vi "HFRR ADV v09 new software.vi"() -> ()   [LabVIEW 2025] (continued)
            n3576 = local read "SEN.RUN HRS"() -> (w4464:dbl)
            n3577 = Divide(x=w4468, y=w4476) -> (x/y=w4475:dbl)
            n3578 = Increment(x=w4475) -> (x+1=w4471:dbl)
            n3579 = Number To Decimal String(number=w4471) -> (decimal integer string=→"run hrs":string)  [unwired: 1 in]
            n3580 = Divide(x=w4464, y=3600.0 ("f")) -> (x/y=w4459:dbl)
            n3581 = Round To Nearest(number=w4459) -> (nearest integer value=w4457:dbl)
            n3582 = Number To Decimal String(number=w4457) -> (decimal integer string=w4458:string)  [unwired: 1 in]
            n3583 = Number To Decimal String(number=w4466) -> (decimal integer string=w4467:string)  [unwired: 1 in]
            n3584 = local read "Model No"() -> (w4472:string)
            n3585 = local read "UUID"() -> (w4567:string)
            n3586 = local read "Serial No"() -> (w4571:string)
            n3587 = local read "Secret Key"() -> (w4572:string)
            n3588 = Concatenate Strings("\",\"MachineSerialNumber\":\"" ("string"), w4571) -> (w4575:string)
            n3589 = Concatenate Strings("\",\"ModelNumber\":\"" ("string"), w4472) -> (w4473:string)
            n3590 = Concatenate Strings("\",\"MachineRuntimeHours\":\"" ("string"), w4458) -> (w4576:string)
            n3591 = Concatenate Strings("\",\"MachineRuntimeCycles\":\"", w4467) -> (w4569:string)
            n3592 = Concatenate Strings(w4525, w4521) -> (w4555:string)
            n3593 = Concatenate Strings(w4524, w4511) -> (w4556:string)
            n3594 = Concatenate Strings(w4523, w4493) -> (w4554:string)
            n3595 = Concatenate Strings(w4575, w4473, w4576, w4569) -> (w4578:string)
            n3596 = Concatenate Strings(w4525, w4520) -> (w4552:string)
            n3597 = Concatenate Strings(w4524, w4510) -> (w4551:string)
            n3598 = Concatenate Strings(w4523, w4492) -> (w4553:string)
            n3599 = Concatenate Strings(w4525, w4519) -> (w4547:string)
            n3600 = Concatenate Strings(w4524, w4509) -> (w4548:string)
            n3601 = Concatenate Strings(w4523, w4491) -> (w4546:string)
            n3602 = Concatenate Strings(w4525, w4518) -> (w4544:string)
            n3603 = Concatenate Strings(w4524, w4508) -> (w4543:string)
            n3604 = Concatenate Strings(w4523, w4490) -> (w4545:string)
            n3605 = Concatenate Strings(w4555, w4556, w4554) -> (w4557:string)
            n3606 = Concatenate Strings(w4525, w4517) -> (w4534:string)
            n3607 = Concatenate Strings(w4524, w4507) -> (w4535:string)
            n3608 = Concatenate Strings(w4525, w4516) -> (w4531:string)
            n3609 = Concatenate Strings(w4524, w4506) -> (w4530:string)
            n3610 = Concatenate Strings(w4523, w4489) -> (w4533:string)
            n3611 = Concatenate Strings(w4523, w4488) -> (w4532:string)
            n3612 = Concatenate Strings("{\"SecretKey\":\"", w4572, w4578, "\",\"UUID\" : \"", w4567, "\",\"SensorInformation\":", "[{" ("string")) -> (w4505:string)
            n3613 = Concatenate Strings(w4552, w4551, w4553) -> (w4550:string)
            n3614 = Concatenate Strings(w4547, w4548, w4546) -> (w4549:string)
            n3615 = Concatenate Strings(w4544, w4543, w4545) -> (w4542:string)
            n3616 = Concatenate Strings(w4534, w4535, w4533) -> (w4536:string)
            n3617 = Concatenate Strings(w4531, w4530, w4532) -> (w4529:string)
            n3618 = Concatenate Strings(w4528, w4540, w4557, w4498) -> (w4504:string)
            n3619 = Concatenate Strings(w4528, w4539, w4550, w4498) -> (w4503:string)
            n3620 = Concatenate Strings(w4528, w4538, w4549, w4498) -> (w4502:string)
            n3621 = Concatenate Strings(w4528, w4537, w4542, w4498) -> (w4501:string)
            n3622 = Concatenate Strings(w4528, w4527, w4536, w4498) -> (w4500:string)
            n3623 = Concatenate Strings(w4528, w4526, w4529, "\"}" ("string")) -> (w4499:string)
            n3624 = Concatenate Strings(w4505, w4504, w4503, w4502, w4501, w4500, w4499, "]}" ("string")) -> (w4496:string)
            n3625 = local read "SEN.RUN HRS"() -> (w4463:dbl)
            n3626 = disable-structure shown="Disabled" {
              frame Disabled {
                n3627 = local read "state"() -> (w4582:string[])
                n3628 = Delete From Array(array=w4582, index=0) -> (array with subset deleted=w4580:string[])  [unwired: 1 in, 1 out]
                n3629 = for {
                  N: 6 -> [_]
                  tunnel: w4580 -> [w4593] mode=indexing
                  tunnel: [w4592] -> w4579 mode=indexing
                  n3630 = Equal?(x=w4593, y="Warning") -> (x = y?=w4589:bool)
                  n3631 = Equal?(x=w4593, y="Healthy") -> (x = y?=w4586:bool)
                  n3632 = Select(t="2" ("y"), s=w4589, f="3" ("y")) -> (s? t:f=w4584:string)
                  n3633 = Select(t="1" ("y"), s=w4586, f=w4584) -> (s? t:f=w4592:string)
                }
                "state1" <- w4579
              }
              frame Enabled {
              }
            }
            n3634 = stacked-sequence {
              tunnel: w4496 -> [w4604 _ _]
              tunnel: [_ _ w4620] -> _
              frame #0 {
                (unwired) FALSE ("convert eol (F)")
                w4606 = enum16{"start", "end", "current"}."start" ("pos mode (0:2)")
                n3635 = local read "Path"() -> (w4600:path)
                n3636 = Path To String(path=w4600) -> (string=w4612:string)
                n3637 = Concatenate Strings(w4612, "\\", "Sensor File Name") -> (w4613:string)
                n3638 = local write "standard output 2"(" ") -> ()
                n3639 = String To Path(string=w4613) -> (path=w4603:path)
                n3640 = call <vilib>:"Open_Create_Replace File.vi"("advisory dialog? (display:T)"=FALSE, "function (open:0)"=T31."create or replace", "file path"=w4603) -> ("error out"=w4616:errorcluster, "refnum"=w4615:refnum<file>)  [unwired: 5 in, 2 out]
                n3641 = Set File Position(refnum=w4615, from (0:start)=w4606, error in=w4616) -> (refnum out=w4596:refnum<file>, error out=w4595:errorcluster)  [unwired: 1 in]
                n3642 = Write to Binary File(file (use dialog)=w4596, data=" ", error in=w4595, 5:FALSE ("prepend array or string size? (T)")) -> (refnum out=w4607:refnum<file>, error out=w4608:errorcluster)  [unwired: 2 in, 1 out]
                n3643 = Set File Position(offset (in bytes) (0)=w4606, refnum=w4607, error in=w4608) -> (refnum out=w4599:refnum<file>, error out=w4598:errorcluster)  [unwired: 1 in]
                n3644 = Write to Binary File(file (use dialog)=w4599, data=w4604, error in=w4598, 5:FALSE ("prepend array or string size? (T)")) -> (error out=w4602:errorcluster)  [unwired: 2 in, 2 out]
                n3645 = flat-sequence {
                  tunnel: w4603 -> [w4618]
                  tunnel: w4602 -> [_]
                  frame #0 {
                    n3646 = call <vilib>:"Read Characters From File.vi"("file path (dialog if empty)"=w4618) -> ("character string"=→"Sensor Health JSON string":string)  [unwired: 5 in, 3 out]
                  }
                }
                "SinglePoint  2" <- w4604
              }
              frame #1 {
              }
              frame #2 {
                (unwired) "\"Stored\": true" ("string")
                n3647 = call <vilib>:"System Exec.vi"("run minimized? (F)"=TRUE, "wait until completion? (T)"=TRUE, "working directory"=path "C:/LAB-IQ-NXT", "command line"="C:\\LAB-IQ-NXT\\JPostH.bat") -> ("standard error"=→"Respose From Server 2":string, "standard output"=w4623:string)  [unwired: 4 in, 2 out]
                "standard output 2" <- w4623
                n3648 = Match Pattern(string=w4623, regular expression="JSONH Check String") -> (match substring=w4621:string, offset past match=w4620:i32)  [unwired: 1 in, 2 out]
                n3649 = Equal?(x=w4621, y="JSONH Check String") -> (x = y?=→"Upload \nConfirmed 2":bool)
              }
            }
            n3650 = Divide(x=w4463, y=3600.0 ("f")) -> (x/y=w4456:dbl)
            n3651 = local read "run time"() -> (w4513:string[])
            n3652 = Round To Nearest(number=w4456) -> (nearest integer value=w4455:dbl)
            n3653 = Number To Decimal String(number=w4455) -> (decimal integer string=w4454:string)  [unwired: 1 in]
            n3654 = Index Array(array="Sensor Information", index (col) #1=0 ("disabled index (col)"), index (col) #2=1 ("index (col)"), index (col) #3=2 ("index (col)"), index (col) #4=3 ("index (col)")) -> (element #1=→"Sensor name":string[], element #2=→"model num":string[], element #3=→"run time":string[], element #4=→"state":string[])  [unwired: 4 in]
            n3655 = Insert Into Array(array=w4513, index=1, new element #1=w4454, new element #2=w4454, new element #3=w4454, new element #4=w4454, new element #5=w4454, new element #6=w4454) -> (w4478:string[])
            "run" <- w4478
            n3656 = local read "out"() -> (w4460:string[])
            n3657 = local read "Sensor Information"() -> (w4480:string[][])
            n3658 = Replace Array Subset(array=w4480, new element #1=w4478, index (col) #1=2 ("disabled index (col)"), new element #2=w4460, index (col) #2=3 ("index (col)")) -> (w4479:string[][])  [unwired: 2 in]
            n3659 = local write "Sensor Information"(w4479) -> ()
          }
        }
        n3660 = case shown="True" w4427 {
          frame False {
          }
          frame True {
            n3661 = Equal?(x="FLAG", y=0.0) -> (x = y?=w4444:bool)
            n3662 = case shown="False" w4444 {
              frame False {
                n3663 = Get Date/Time In Seconds() -> (seconds since 1Jan1904=w4450:timestamp)
                n3664 = local read "START 2"() -> (w4448:dbl)
                n3665 = To Double Precision Float(number=w4450) -> (double precision float=w4449:dbl)
                n3666 = Subtract(x=w4449, y=w4448) -> (x-y=→"SENSOR TIME  2":dbl)
              }
              frame True {
                n3667 = Get Date/Time In Seconds() -> (seconds since 1Jan1904=w4452:timestamp)
                n3668 = To Double Precision Float(number=w4452) -> (double precision float=→"START 2":dbl)
                n3669 = local write "FLAG"(100.0 ("FLAG")) -> ()
              }
            }
          }
        }
        n3670 = disable-structure shown="Disabled" {
          disable-tunnel: w4430 -> [w4439 _]
          disable-tunnel: [w4438 _] -> w4429
          frame Disabled {
            n3671 = local read "Json St Flg"() -> (w4437:bool)
            n3672 = case shown="True" w4437 {
              tunnel: w4439 -> [w4440 w4442]
              tunnel: [w4440 w4441] -> w4438
              frame False {
              }
              frame True {
                n3673 = Increment(x=w4442) -> (x+1=w4441:dbl)
                "T cycle" <- w4441
                n3674 = local write "Json St Flg"(FALSE ("Json St Flg")) -> ()
              }
            }
          }
          frame Enabled {
          }
        }
        n3675 = local read "Quit"() -> (w4424:bool)
      }
    }
    frame Enabled {
    }
  }
  n3676 = stacked-sequence {
    tunnel: [w4822] -> w38
    frame #0 {
      w4822 = FALSE ("Upload \nConfirmed")
      n3677 = local write "Upload \nConfirmed"(w4822) -> ()
      n3678 = local write "St Str"("") -> ()
    }
  }
  n3679 = disable-structure shown="Disabled" {
    disable-tunnel: w38 -> [w4823 _]
    frame Disabled {
      n3680 = case shown="True" {
        selector: _ -> [_ _]
        tunnel: w4823 -> [_ w4824]
        frame False {
        }
        frame True {
          n3681 = while {
            tunnel: [w4830] -> _
            tunnel: w4824 -> [_]
            i -> [w4830]
            stop <- w4825 stop-if-true
            n3682 = local read "Json End Flg"() -> (w4829:bool)
            n3683 = Wait (ms)(milliseconds to wait=u32 20 ("Refresh Rate (ms)")) -> ()  [unwired: 1 out]
            n3684 = local read "refresh flag"() -> (w4826:bool)
            n3685 = local read "RUN"() -> (w4827:bool)
            n3686 = And(x=w4827, y=w4826) -> (x .and. y?=w4828:bool)
            n3687 = Or(x=w4828, y=w4829) -> (x .or. y?=w4831:bool)
            "AR Led" <- w4831
            n3688 = case shown="True" w4831 {
              frame False {
              }
              frame True {
                w4848 = "\",\""
                n3689 = local read "UUID"() -> (w4846:string)
                n3690 = local write "refresh flag"(FALSE ("refresh flag")) -> ()
                n3691 = local read "time"() -> (w4835:dbl)
                n3692 = Multiply(x=w4835, y=60.0) -> (x*y=w4834:dbl)
                n3693 = Concatenate Strings("UUID\" : \"", w4846, "\"}") -> (w4849:string)
                n3694 = Number To Fractional String(number=w4834, width (-)=i16 10, precision (6)=i16 4) -> (F-format string=w4863:string)  [unwired: 1 in]
                n3695 = Concatenate Strings("{", "\"Time\":\"", w4863, w4848) -> (w4858:string)
                n3696 = stacked-sequence {
                  tunnel: w4848 -> [w4911 w4919 w4926 w4934 w4942 w4951 w4958]
                  tunnel: [w4912 _ _ _ _ _ _] -> w4862
                  tunnel: [_ w4920 _ _ _ _ _] -> w4861
                  tunnel: [_ _ w4927 _ _ _ _] -> w4860
                  tunnel: [_ _ _ w4936 _ _ _] -> w4859
                  tunnel: w4849 -> [_ _ _ _ _ _ w4969]
                  tunnel: [_ _ _ _ _ _ w4968] -> w4845
                  tunnel: [_ _ _ _ _ w4948 _] -> w4844
                  tunnel: [_ _ _ _ w4941 _ _] -> w4843
                  frame #0 {
                    n3697 = local read "NORMAL LOAD"() -> (w4910:dbl)
                    n3698 = Number To Fractional String(number=w4910, width (-)=i16 10, precision (6)=i16 4) -> (F-format string=w4913:string)  [unwired: 1 in]
                    n3699 = Concatenate Strings("NormalLoad\":\"", w4913, w4911) -> (w4912:string)
                  }
                  frame #1 {
                    n3700 = local read "Temp"() -> (w4918:dbl)
                    n3701 = Number To Fractional String(number=w4918, width (-)=i16 10, precision (6)=i16 4) -> (F-format string=w4921:string)  [unwired: 1 in]
                    n3702 = Concatenate Strings("Temperature\":\"", w4921, w4919) -> (w4920:string)
                  }
                  frame #2 {
                    n3703 = local read "cof"() -> (w4924:dbl)
                    n3704 = Number To Fractional String(number=w4924, width (-)=i16 10, precision (6)=i16 4) -> (F-format string=w4928:string)  [unwired: 1 in]
                    n3705 = Concatenate Strings("FrictionalForce\":\"", w4928, w4926) -> (w4927:string)
                  }
                  frame #3 {
                    n3706 = local read "Set Hz"() -> (w4932:dbl)
                    n3707 = Multiply(x=w4932, y=60.0) -> (x*y=w4931:dbl)
                    n3708 = Number To Fractional String(number=w4931, width (-)=i16 10, precision (6)=i16 4) -> (F-format string=w4937:string)  [unwired: 1 in]
                    n3709 = Concatenate Strings("Speed\":\"", w4937, w4934) -> (w4936:string)
                  }
                  frame #4 {
                    n3710 = local read item#-1() -> (w4940)
                    n3711 = Number To Fractional String(number=w4940, width (-)=i16 10, precision (6)=i16 4) -> (F-format string=w4944:string)  [unwired: 1 in]
                    n3712 = Concatenate Strings("LinearDeformation\":\"", w4944, w4942) -> (w4941:string)
                  }
                  frame #5 {
                    n3713 = local read "AIR TEMP"() -> (w4947:dbl)
                    n3714 = local read "Json St Flg"() -> (w4949:bool)
                    n3715 = local read "Json End Flg"() -> (w4950:bool)
                    n3716 = Number To Fractional String(number=w4947, width (-)=i16 10, precision (6)=i16 4) -> (F-format string=w4953:string)  [unwired: 1 in]
                    n3717 = Concatenate Strings("Vibration\":\"", w4953, w4951) -> (w4948:string)
                    n3718 = And(x=w4949, y=w4950) -> ()  [unwired: 1 out]
                  }
                  frame #6 {
                    n3719 = local read "Json End Flg"() -> (w4957:bool)
                    n3720 = Get Date/Time In Seconds() -> (seconds since 1Jan1904=w4965:timestamp)
                    n3721 = local read "Json St Flg"() -> (w4956:bool)
                    n3722 = To Double Precision Float(number=w4965) -> (double precision float=w4964:dbl)
                    n3723 = Subtract(x=w4964, y=2082844800.0) -> (x-y=w4962:dbl)
                    n3724 = Number To Fractional String(number=w4962, width (-)=i16 12, precision (6)=i16 0) -> (F-format string=w4959:string)  [unwired: 1 in]
                    n3725 = case shown="True" w4957 {
                      tunnel: ["" w4972] -> w4966
                      tunnel: w4959 -> [_ w4973]
                      tunnel: w4958 -> [_ w4971]
                      frame False {
                      }
                      frame True {
                        n3726 = local write "Json End Flg"(FALSE ("Json St Flg")) -> ()
                        n3727 = Concatenate Strings("End\": \"", w4973, w4971) -> (w4972:string)
                      }
                    }
                    n3728 = case shown="True" w4956 {
                      tunnel: [w4976 w4979] -> w4967
                      tunnel: w4959 -> [_ w4980]
                      tunnel: w4958 -> [_ w4977]
                      frame False {
                        n3729 = local read "St Str"() -> (w4976:string)
                      }
                      frame True {
                        n3730 = Concatenate Strings("Start\":\"", w4980, w4977) -> (w4979:string)
                        "St Str" <- w4979
                        n3731 = local write "Json St Flg"(FALSE ("Json St Flg")) -> ()
                      }
                    }
                    n3732 = Concatenate Strings(w4967, w4966, w4969) -> (w4968:string)
                  }
                }
                n3733 = local read "FILE"() -> (w4837:string)
                n3734 = Concatenate Strings("\",\"OperatorID\":\"" ("string"), "Operator ID") -> (w4840:string)
                n3735 = Concatenate Strings("\",\"DatasetTitle\":\"" ("string"), w4837) -> (w4839:string)
                n3736 = Concatenate Strings("\",\"SerialNumber\":\"" ("string"), "Serial No") -> (w4869:string)
                n3737 = Concatenate Strings("\",\"ModelNumber\":\"" ("string"), "Model No") -> (w4868:string)
                n3738 = Concatenate Strings(w4869, w4868) -> (w4851:string)
                n3739 = Concatenate Strings("{\"SecretKey\":\"", "Secret Key", w4851, w4840, w4839, "\",\"Samples\":[") -> (w4856:string)
                n3740 = Concatenate Strings(w4858, w4862, w4861, w4860, w4859, w4843, w4844, w4845) -> (w4857:string)
                n3741 = Concatenate Strings(w4856, w4857, "]}") -> (w4855:string)
                n3742 = stacked-sequence {
                  tunnel: w4855 -> [w4884 _ _]
                  tunnel: [_ _ w4901] -> _
                  frame #0 {
                    (unwired) FALSE ("convert eol (F)")
                    w4886 = enum16{"start", "end", "current"}."start" ("pos mode (0:2)")
                    n3743 = Path To String(path="Path") -> (string=w4892:string)
                    n3744 = Concatenate Strings(w4892, "\\", "Data File Name") -> (w4894:string)
                    n3745 = local write "standard output"(" ") -> ()
                    n3746 = String To Path(string=w4894) -> (path=w4883:path)
                    n3747 = call <vilib>:"Open_Create_Replace File.vi"("advisory dialog? (display:T)"=FALSE, "function (open:0)"=T31."create or replace", "file path"=w4883) -> ("error out"=w4897:errorcluster, "refnum"=w4896:refnum<file>)  [unwired: 5 in, 2 out]
                    n3748 = Set File Position(refnum=w4896, from (0:start)=w4886, error in=w4897) -> (refnum out=w4877:refnum<file>, error out=w4876:errorcluster)  [unwired: 1 in]
                    n3749 = Write to Binary File(file (use dialog)=w4877, data=" ", error in=w4876, 5:FALSE ("prepend array or string size? (T)")) -> (refnum out=w4887:refnum<file>, error out=w4888:errorcluster)  [unwired: 2 in, 1 out]
                    n3750 = Set File Position(offset (in bytes) (0)=w4886, refnum=w4887, error in=w4888) -> (refnum out=w4880:refnum<file>, error out=w4879:errorcluster)  [unwired: 1 in]
                    n3751 = Write to Binary File(file (use dialog)=w4880, data=w4884, error in=w4879, 5:FALSE ("prepend array or string size? (T)")) -> (error out=w4882:errorcluster)  [unwired: 2 in, 2 out]
                    n3752 = flat-sequence {
                      tunnel: w4883 -> [w4899]
                      tunnel: w4882 -> [_]
                      frame #0 {
                        n3753 = call <vilib>:"Read Characters From File.vi"("file path (dialog if empty)"=w4899) -> ("character string"=→"JSON string":string)  [unwired: 5 in, 3 out]
                      }
                    }
                    "SinglePoint" <- w4884
                  }
                  frame #1 {
                  }
                  frame #2 {
                    (unwired) "\"Stored\": true" ("string")
                    n3754 = call <vilib>:"System Exec.vi"("run minimized? (F)"=TRUE, "wait until completion? (T)"=TRUE, "working directory"=path "C:/LAB-IQ-NXT", "command line"="C:\\LAB-IQ-NXT\\JPost.bat") -> ("standard error"=→"Respose From Server":string, "standard output"=w4904:string)  [unwired: 4 in, 2 out]
                    "standard output" <- w4904
                    n3755 = Match Pattern(string=w4904, regular expression="JSON Check String") -> (match substring=w4902:string, offset past match=w4901:i32)  [unwired: 1 in, 2 out]
                    n3756 = Equal?(x=w4902, y="JSON Check String") -> (x = y?=→"Upload \nConfirmed":bool)
                  }
                }
              }
            }
            n3757 = local read "Quit"() -> (w4825:bool)
          }
        }
      }
    }
    frame Enabled {
    }
  }
  n3758 = disable-structure shown="Disabled" {
    disable-tunnel: _ -> [w4987 _]
    frame Disabled {
      n3759 = while {
        shift-right: [w4995] -> w4983
        shift-left: _ -> [w4996]
        shift-right: [w4993] -> w4984
        shift-left: errorcluster {"status"=TRUE, "code"=0, "source"="Init"} ("error out") -> [w4994]
        shift-right: [w4991] -> _
        shift-left: "" -> [w4992]
        tunnel: [w4989] -> _
        tunnel: w4987 -> [_]
        i -> [w4989]
        stop <- w4988 stop-if-true
        n3760 = flat-sequence {
          tunnel: [w4997] -> w4990
          frame #0 {
            n3761 = Wait (ms)(milliseconds to wait=10.0 ("Delay")) -> (millisecond timer value=w4997:u32)
          }
        }
        n3762 = case shown="No Error" w4994 {
          selector: w4994 -> [w5027 w5146]
          tunnel: [w5010 w5148] -> w4995
          tunnel: [w5009 w5147] -> w4993
          tunnel: w4996 -> [w5028 w5140]
          tunnel: w4992 -> [w5008 w5139]
          tunnel: [w5007 w5139] -> w4991
          tunnel: w4990 -> [_ _]
          frame No Error {
            n3763 = Concatenate Strings("\r", "\n") -> (w5019:string)  [unwired: 1 in]
            n3764 = case shown="True" w5020 {
              tunnel: w5028 -> [w5052 w5059]
              tunnel: w5027 -> [w5051 w5058]
              tunnel: [w5052 w5057] -> w5026
              tunnel: [w5051 w5056] -> w5006
              tunnel: w5019 -> [_ w5055]
              frame False {
              }
              frame True {
                n3765 = VISA Write(VISA resource name=w5059, write buffer=w5055, error in (no error)=w5058) -> (VISA resource name out=w5057:refnum<visa-resource-name>, error out=w5056:errorcluster)  [unwired: 1 out]
                n3766 = local write "Read String"("") -> ()
                n3767 = local write item#-1(FALSE) -> ()
              }
            }
            n3768 = property class="Instr"(reference=w5026, error in=w5006) -> (reference out=w5025:refnum<visa-resource-name>, error out=w5024:errorcluster, "Serial Settings:Number of Bytes at Serial Port"=w5023:u32)
            n3769 = Greater?(x=w5023, y=u32 100) -> (0:w5021:bool)
            n3770 = case shown="True" w5021 {
              tunnel: w5025 -> [w5062 w5086]
              tunnel: w5024 -> [w5061 w5085]
              tunnel: w5023 -> [_ w5084]
              tunnel: [w5062 w5083] -> w5012
              tunnel: [w5061 w5082] -> w5011
              tunnel: w5008 -> [w5060 w5081]
              tunnel: [w5060 ""] -> w5007
              frame False {
              }
              frame True {
                w5071 = u32 6 ("y")
                # "Page 84 of \nmanual"
                n3771 = VISA Read(VISA resource name=w5086, byte count=w5084, error in (no error)=w5085) -> (VISA resource name out=w5083:refnum<visa-resource-name>, read buffer=w5079:string, error out=w5082:errorcluster)  [unwired: 1 out]
                n3772 = while {
                  tunnel: w5079 -> [w5135]
                  tunnel: [w5131] -> w5073 mode=indexing
                  tunnel: [w5125] -> w5077 mode=indexing
                  tunnel: [w5123] -> _
                  i -> [w5123]
                  stop <- w5128 stop-if-true
                  n3773 = String Subset(string=w5135, offset (0)=w5123) -> (substring=w5130:string)  [unwired: 1 in]
                  n3774 = String To Byte Array(string=w5130) -> (unsigned byte array=w5134:u8[])
                  n3775 = String Length(string=w5130) -> (length=w5129:i32)
                  n3776 = Index Array(array=w5134) -> (element=w5133:u8)  [unwired: 1 in]
                  n3777 = Equal To 0?(x=w5129) -> (x = 0?=w5128:bool)
                  n3778 = Number To Boolean Array(number=w5133) -> (Boolean array=w5127:bool[])
                  n3779 = Reverse 1D Array(array=w5127) -> (reversed array=w5126:bool[])
                  n3780 = And(x=w5127, y=bool[] [FALSE, FALSE, FALSE, FALSE, FALSE, FALSE, TRUE, TRUE] ("Boolean array")) -> (x .and. y?=w5131:bool[])
                  n3781 = And(x=w5126, y=bool[] [FALSE, FALSE, TRUE, TRUE, TRUE, TRUE, TRUE, TRUE] ("Boolean array")) -> (x .and. y?=w5125:bool[])
                }
                n3782 = Concatenate Strings(w5081, w5079) -> (→"Read String":string)
                n3783 = while {
                  tunnel: w5073 -> [w5122] mode=indexing
                  tunnel: [w5118] -> w5076
                  i -> [w5118]
                  stop <- w5119 stop-if-true
                  n3784 = Search 1D Array(1D array=w5122, element=TRUE) -> (index of element=w5120:i32)  [unwired: 1 in]
                  n3785 = Less Than 0?(x=w5120) -> (x < 0?=w5119:bool)
                }
                n3786 = Delete From Array(array=w5077, length=w5076, index (row)=0) -> (array with subset deleted=w5072:bool[][])  [unwired: 1 in, 1 out]
                n3787 = Array Size(array=w5072) -> (size(s)=w5074:i32[])
                n3788 = Index Array(array=w5074) -> (element=w5066:i32)  [unwired: 1 in]
                n3789 = Greater?(x=w5066, y=w5071) -> (0:w5069:bool)
                n3790 = Subtract(x=w5066, y=w5071) -> (x-y=w5070:u32)
                n3791 = Select(t=w5070, s=w5069, f=u32 0) -> (s? t:f=w5067:u32)
                n3792 = while {
                  tunnel: w5072 -> [w5105]
                  tunnel: [w5107] -> w5065 mode=indexing
                  tunnel: w5067 -> [w5089]
                  i -> [w5106]
                  stop <- w5104 stop-if-true
                  w5096 = 6 ("index")
                  w5095 = 2 ("length")
                  # "Page 65 of \nmanual"
                  n3793 = Multiply(x=u32 3 ("y"), y=w5106) -> (x*y=w5103:u32)
                  n3794 = Divide(x=u32 102 ("y"), y=u32 65520) -> (x/y=w5113:dbl)
                  n3795 = Greater Or Equal?(x=w5103, y=w5089) -> (x >= y?=w5104:bool)
                  n3796 = Index Array(array=w5105, index (row) #1=w5103) -> (element #1=w5101:bool[], element #2=w5100:bool[], element #3=w5099:bool[])  [unwired: 5 in]
                  n3797 = Reverse 1D Array(array=w5101) -> (reversed array=w5094:bool[])
                  n3798 = Reverse 1D Array(array=w5100) -> (reversed array=w5098:bool[])
                  n3799 = Reverse 1D Array(array=w5099) -> (reversed array=w5097:bool[])
                  n3800 = Delete From Array(array=w5094, length=w5095, index=w5096) -> (array with subset deleted=w5090:bool[])  [unwired: 1 out]
                  n3801 = Delete From Array(array=w5098, length=w5095, index=w5096) -> (array with subset deleted=w5091:bool[])  [unwired: 1 out]
                  n3802 = Delete From Array(array=w5097, length=w5095, index=w5096) -> (array with subset deleted=w5092:bool[])  [unwired: 1 out]
                  n3803 = Insert Into Array(array=bool[] [] ("Boolean array"), new element #1=w5090, new element #2=w5091, new element #3=w5092) -> (w5093:bool[])  [unwired: 1 in]
                  n3804 = Boolean Array To Number(Boolean array=w5093) -> (number=w5102:u32)
                  n3805 = Multiply(x=w5113, y=w5102) -> (x*y=w5112:dbl)
                  n3806 = Decrement(x=w5112) -> (x-1=w5111:dbl)
                  n3807 = Divide(x=w5111, y=u32 100) -> (x/y=w5109:dbl)
                  n3808 = Multiply(x=w5109, y=u32 10) -> (x*y=w5107:dbl)
                }
                n3809 = Delete From Array(array=w5065) -> (array with subset deleted=w5064:dbl[])  [unwired: 2 in, 1 out]
                "Waveform Graph 5" <- w5064
                "Waveform Chart 3" <- w5064
                n3810 = call-poly <vilib>:"Mean.vi"("X"=w5064) -> ("mean"=w5063:dbl)  [unwired: 1 out]
                n3811 = case shown="True" {
                  selector: _ -> [_ _]
                  tunnel: w5063 -> [_ w5088]
                  frame False {
                  }
                  frame True {
                    n3812 = local write item#-1(FALSE ("Zero 4")) -> ()
                    "z_measure" <- w5088
                  }
                }
              }
            }
            n3813 = local read item#-1() -> (w5003)
            n3814 = local read item#-1() -> (w5002)
            n3815 = local read item#-1() -> (w5004)
            n3816 = local read item#-1() -> (w5001)
            n3817 = case shown="True" w4999 {
              tunnel: w5003 -> [_ w5031]
              tunnel: w5004 -> [_ w5030]
              frame False {
              }
              frame True {
                n3818 = Build Array(w5031, w5030) -> (w5029:void[])
                n3819 = local read item#-1() -> (w5034)
                n3820 = Build Array (concatenate)(w5034, w5029) -> (w5032:void[])
                n3821 = local write item#-1(w5032) -> ()
                n3822 = local write item#-1(FALSE ("Boolean 8")) -> ()
              }
            }
            n3823 = call "Build XY Graph"("Enable"=w5001, "Reset"=w5002, "Y Input"=w5004, "X Input"=w5003) -> ("XY Graph"=w5000:cluster{"Y":dbl[], "Y":dbl[]}[])  [unwired: 6 in, 1 out]
            n3824 = case shown="True" {
              selector: _ -> [_ _]
              frame False {
              }
              frame True {
                n3825 = local read item#-1() -> (w5035)
                n3826 = Index Array(array=w5035, index (col) #1=0 ("disabled index (col)"), index (col) #2=1 ("index (col)")) -> (element #1=w5037, element #2=w5036)  [unwired: 2 in]
                n3827 = call <vilib>:"Linear Fit.vi"("Y"=w5037, "X"=w5036) -> ()  [unwired: 9 in, 5 out]
                n3828 = local write item#-1(FALSE ("Boolean 9")) -> ()
              }
            }
            n3829 = case shown="True" {
              selector: _ -> [_ _]
              frame False {
              }
              frame True {
                n3830 = local write item#-1(dbl[][] [] ("Captured Values")) -> ()
                n3831 = local write item#-1(FALSE ("Boolean 7")) -> ()
              }
            }
            n3832 = Concatenate Strings("\r", "\n") -> (w5014:string, w5013:string)
            n3833 = case shown="True" w5005 {
              tunnel: w5012 -> [w5044 w5050]
              tunnel: w5011 -> [w5043 w5049]
              tunnel: [w5044 w5048] -> w5010
              tunnel: [w5043 w5047] -> w5009
              tunnel: w5014 -> [_ w5046]
              frame False {
              }
              frame True {
                n3834 = VISA Write(VISA resource name=w5050, write buffer=w5046, error in (no error)=w5049) -> (VISA resource name out=w5048:refnum<visa-resource-name>, error out=w5047:errorcluster)  [unwired: 1 out]
                n3835 = local write item#-1(FALSE ("WRITE")) -> ()
              }
            }
          }
          frame Error {
            w5138 = u16 10 items=["1.0"=10, "1.5"=15, "2.0"=20] ("stop bits (10: 1 bit)")
            n3836 = Wait (ms)(milliseconds to wait=u32 20) -> ()  [unwired: 1 out]
            n3837 = VISA Close(VISA resource name=w5140, error in (no error)=w5146) -> (error out=w5145:errorcluster)
            n3838 = call <vilib>:"Clear Errors.vi"("error in (no error)"=w5145) -> ("error out"=w5144:errorcluster)  [unwired: 5 in, 1 out]
            n3839 = call-poly "VISA Configure Serial Port"("timeout (10sec)"=u32 200, "Enable Termination\nChar (T)"=TRUE ("Enable Termination\nChar (T)"), "baud rate (9600)"=u32 921600, "error in (no error)"=w5144, "stop bits (10: 1 bit)"=w5138) -> ("VISA resource name"=w5136:refnum<visa-resource-name>, "VISA resource name out"=w5148:refnum<visa-resource-name>, "error out"=w5147:errorcluster)  [unwired: 8 in]
          }
        }
        n3840 = local read "Quit"() -> (w4988:bool)
      }
      n3841 = VISA Close(VISA resource name=w4983, error in (no error)=w4984) -> (error out=w4982:errorcluster)
      n3842 = call <vilib>:"Clear Errors.vi"("error in (no error)"=w4982) -> ()  [unwired: 5 in, 2 out]
    }
    frame Enabled {
    }
  }
  n3843 = disable-structure shown="Disabled" {
    disable-tunnel: _ -> [w5153 _]
    frame Disabled {
      n3844 = while {
        tunnel: [w5160] -> _
        shift-right: [w5157] -> w5150
        shift-left: _ -> [w5159]
        shift-right: [w5158] -> w5151
        shift-left: errorcluster {"status"=TRUE, "code"=0, "source"="Init"} ("error out") -> [w5156]
        tunnel: w5153 -> [_]
        i -> [w5160]
        stop <- w5154 stop-if-true
        n3845 = flat-sequence {
          tunnel: w5156 -> [w5251]
          tunnel: [w5251] -> w5155
          frame #0 {
            n3846 = Wait (ms)(milliseconds to wait=u32 50) -> ()  [unwired: 1 out]
          }
        }
        n3847 = case shown="No Error" w5155 {
          selector: w5155 -> [w5201 w5244]
          tunnel: w5159 -> [w5200 w5243]
          tunnel: [w5167 w5234] -> w5158
          tunnel: [w5168 w5242] -> w5157
          frame No Error {
            w5194 = T32 {"Mode"=enum."RTU", "Slave Address"=1} ("Serial Parameters")
            n3848 = call-poly <vilib>:"MB Serial Master Query (poly).vi"("VISA resource name"=w5200, "Starting Address"=i16 1000, "Quantity"=u16 1, "Timeout"=u32 1000, "error in"=w5201, "Serial Parameters"=w5194) -> ("VISA resource name out"=w5195:refnum<visa-resource-name>, "Input Registers"=w5197:u16[], "error out"=w5193:errorcluster)  [unwired: 10 in, 1 out]
            n3849 = Random Number (0-1)() -> (number: 0 to 1=w5182:dbl)
            n3850 = Index Array(array=w5197, index=0) -> (element=w5192:u16)
            n3851 = Subtract(x=w5182, y=0.5) -> (x-y=w5181:dbl)
            n3852 = Divide(x=w5192, y=10 ("index")) -> (x/y=w5186:dbl)
            n3853 = Multiply(x=w5181, y=0.5) -> (x*y=w5180:dbl)
            n3854 = Add(x=w5186, y=w5180) -> (x+y=w5185:dbl)
            n3855 = local read "Amb temp"() -> (w5169:dbl)
            n3856 = Multiply(x=w5185, y=0.2) -> (x*y=w5189:dbl)
            n3857 = Multiply(x=w5169, y=0.8) -> (x*y=w5187:dbl)
            n3858 = Add(x=w5189, y=w5187) -> (x+y=w5170:dbl)
            n3859 = local read "set temp old"() -> (w5164:dbl)
            n3860 = local write "Amb temp"(w5170) -> ()
            n3861 = Select(t="SetTemp 2", s="Heater", f=100.0) -> (s? t:f=w5165:dbl)
            n3862 = Not Equal?(x=w5165, y=w5164) -> (x != y?=w5163:bool)
            n3863 = case shown="True" w5163 {
              tunnel: w5195 -> [w5229 w5231]
              tunnel: [w5228 w5231] -> w5175
              tunnel: w5193 -> [w5227 w5230]
              tunnel: [w5226 w5230] -> w5173
              tunnel: w5165 -> [w5221 _]
              tunnel: w5194 -> [w5223 w5232]
              tunnel: [w5223 w5232] -> w5176
              frame True {
                n3864 = Multiply(x=w5221, y=10 ("index")) -> (x*y=w5220:dbl)
                n3865 = call-poly <vilib>:"MB Serial Master Query (poly).vi"("VISA resource name"=w5229, "Address"=u16 0, "Holding Register"=w5220, "Timeout"=u32 1000, "error in"=w5227, "Serial Parameters"=w5223) -> ("VISA resource name out"=w5228:refnum<visa-resource-name>, "error out"=w5226:errorcluster)  [unwired: 11 in, 1 out]
                "set temp old" <- w5221
              }
              frame False {
              }
            }
            n3866 = flat-sequence {
              tunnel: [w5202] -> _
              tunnel: [w5202] -> w5172
              tunnel: w5173 -> [w5202]
              frame #0 {
                n3867 = Wait (ms)(milliseconds to wait=u32 100) -> ()  [unwired: 1 out]
              }
            }
            n3868 = call "Elapsed Time12"("Time Target (s)"=2.0, "Auto Reset"=TRUE) -> ("Time has Elapsed"=w5177:bool)  [unwired: 10 in, 7 out]
            n3869 = case shown="True" w5177 {
              tunnel: w5176 -> [w5206 w5219]
              tunnel: [w5206 w5219] -> _
              tunnel: [w5205 w5217] -> w5168
              tunnel: w5175 -> [w5205 w5218]
              tunnel: [w5204 w5215] -> w5167
              tunnel: w5172 -> [w5204 w5216]
              frame False {
              }
              frame True {
                n3870 = call-poly <vilib>:"MB Serial Master Query (poly).vi"("VISA resource name"=w5218, "Starting Address"=i16 1003 ("Addr"), "Quantity"=u16 1, "Timeout"=u32 1000, "error in"=w5216, "Serial Parameters"=w5219) -> ("VISA resource name out"=w5217:refnum<visa-resource-name>, "Input Registers"=w5212:u16[], "error out"=w5215:errorcluster)  [unwired: 10 in, 1 out]
                n3871 = Index Array(array=w5212, index=0) -> (element=w5211:u16)
                n3872 = Divide(x=w5211, y=u16 10) -> (x/y=w5207:dbl)
                n3873 = local write "set temp old"(w5207) -> ()
                n3874 = local write "SetTemp"(w5207) -> ()
              }
            }
            "Error Code" <- w5167
            n3875 = Unbundle(w5167) -> ("status"=→"TK4 status":bool)  [unwired: 2 out]
            "SetTemp" <- "SetTemp 2"
          }
          frame Error {
            w5246 = u16 0 items=["None", "Odd", "Even", "Mark", "Space"] ("Parity")
            w5247 = u16 0 items=["None", "XON/XOFF", "RTS/CTS", "XON/XOFF & RTS/CTS", "DTR/DSR", "XON/XOFF & DTR/DSR"] ("Flow Control")
            n3876 = VISA Clear(VISA resource name=w5243, error in (no error)=w5244) -> (VISA resource name out=w5237:refnum<visa-resource-name>, error out=w5235:errorcluster)
            n3877 = VISA Close(VISA resource name=w5237, error in (no error)=w5235) -> (error out=w5236:errorcluster)
            n3878 = call <vilib>:"Clear Errors.vi"("error in (no error)"=w5236) -> ("error out"=w5245:errorcluster)  [unwired: 5 in, 1 out]
            n3879 = Unbundle By Name(T32 {"Mode"=enum."RTU", "Slave Address"=1} ("input cluster")) -> ("Mode"=w5248:enum16{"RTU", "ASCII"})
            n3880 = call <vilib>:"MB Serial Init.vi"("Timeout"=u32 100, "Flow Control"=w5247, "Mode"=w5248, "error in (no error)"=w5245, "Parity"=w5246, "Baud Rate"=u32 9600, "VISA resource name"="Lubrication System COM Port :") -> ("error out"=w5234:errorcluster, "VISA resource name out"=w5242:refnum<visa-resource-name>)  [unwired: 3 in]
            n3881 = local write "set temp old"(0.0 ("set temp old")) -> ()
            n3882 = Unbundle(w5234) -> ("status"=w5233:bool)  [unwired: 2 out]
            n3883 = case shown="True" w5233 {
              selector: w5233 -> [_ w5250]
              frame False {
              }
              frame True {
                n3884 = local write "TK4 status"(w5250) -> ()
              }
            }
          }
        }
        n3885 = local read "Quit"() -> (w5154:bool)
      }
      n3886 = VISA Close(VISA resource name=w5150, error in (no error)=w5151) -> (error out=w5149:errorcluster)
      n3887 = call <vilib>:"Clear Errors.vi"("error in (no error)"=w5149) -> ()  [unwired: 5 in, 2 out]
    }
    frame Enabled {
    }
  }
